vi "RTB.vi"() -> ()   [LabVIEW 2019]
uses:
  <vilib>/Analysis/NI_AALPro.lvlib
  <vilib>/Analysis/NI_AALBase.lvlib
panel:
  out "mean":dbl
  in  "x":dbl=50.0 format="%#_13g"
  out "Lower 2":dbl
  out "Upper 2":dbl
  out "Boolean 3":bool
  out "output array 2":dbl[](array[numeric])
  out "size(s) 2":dbl
  in  "OK Button":bool
  out "Waveform Graph":dbl[](graph)
  out "initialized array":dbl[](array[numeric])
  in  "stop":bool
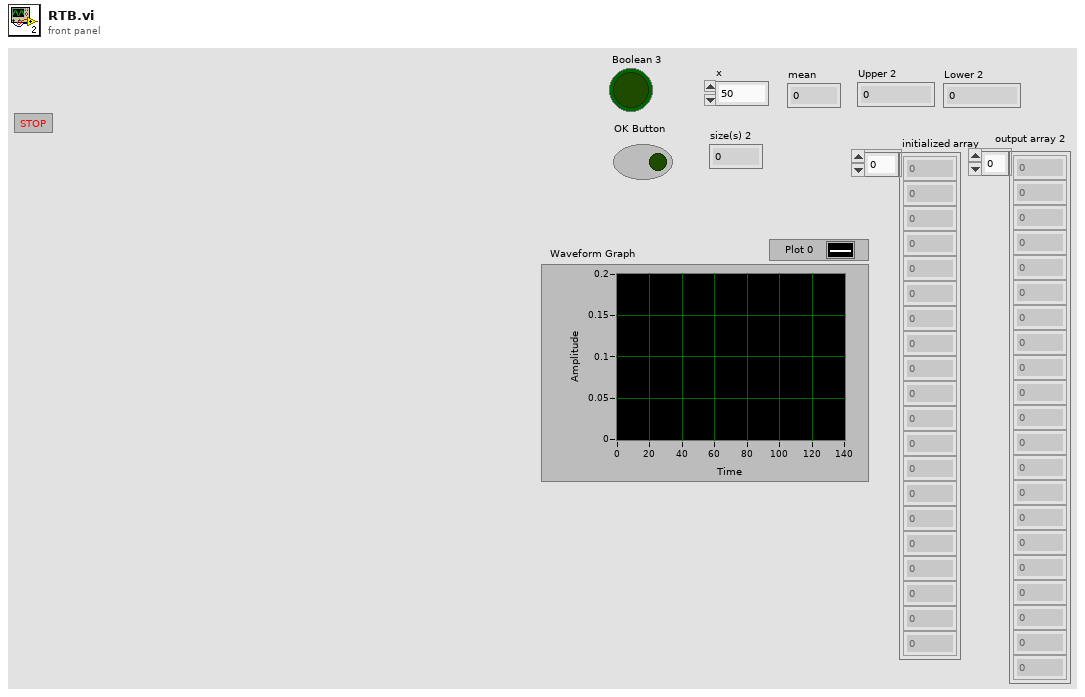
[diagram p1: front panel]
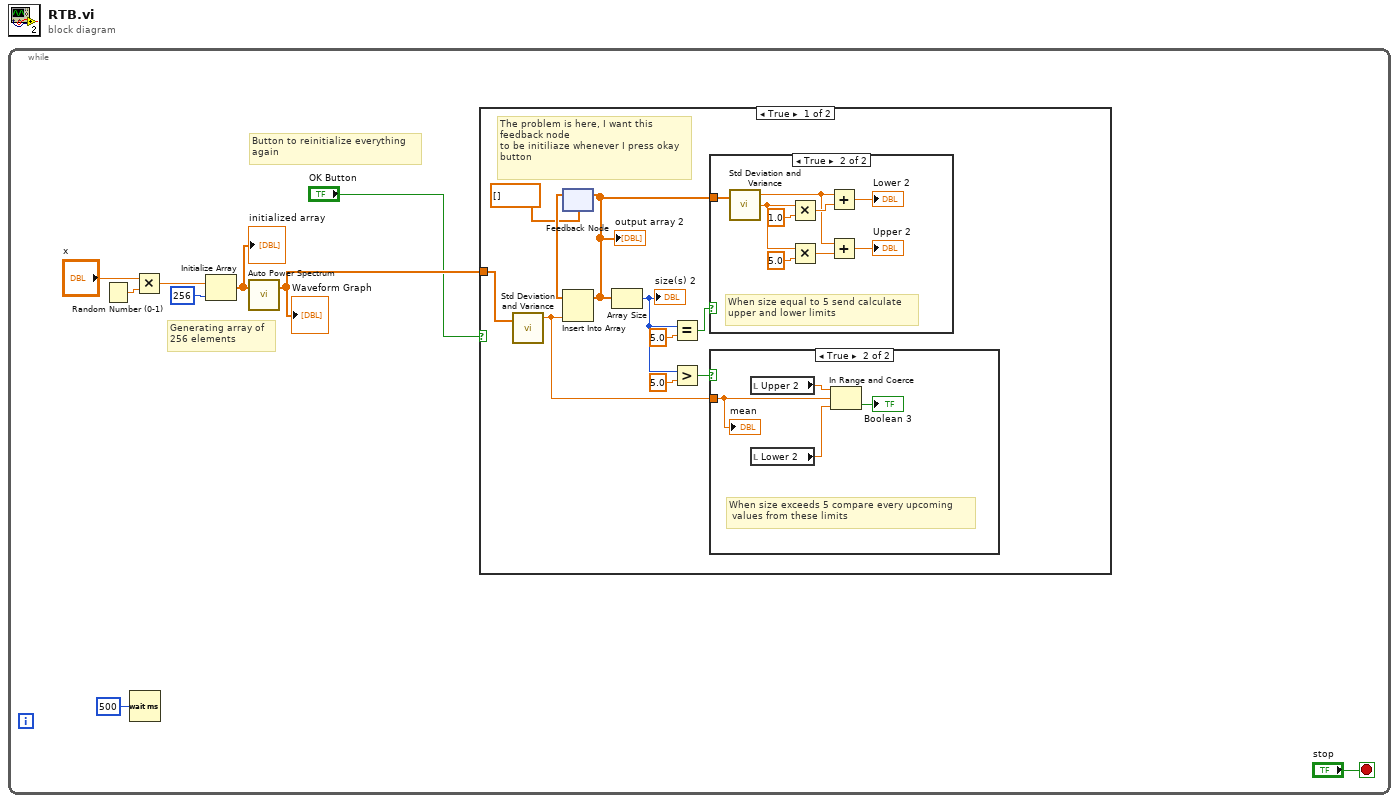
[diagram p0: block diagram]
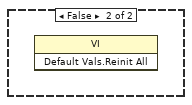
[diagram p4: hidden frame]
diagram:
  n1 = while {
    stop <- "stop" stop-if-true
    # "Generating array of \n256 elements"
    # "Button to reinitialize everything \nagain"
    n2 = Random Number (0-1)() -> (number: 0 to 1=w3:dbl)
    n3 = Wait (ms)(milliseconds to wait=u32 500) -> ()  [unwired: 1 out]
    n4 = Multiply(x="x", y=w3) -> (x*y=w1:dbl)
    n5 = Initialize Array(w1, 256 ("dimension size")) -> (w7:dbl[])
    "initialized array" <- w7
    n6 = call <vilib>:"Auto Power Spectrum.vi"("Signal (V)"=w7) -> ("Power Spectrum (V^2 rms)"=w6:dbl[])  [unwired: 1 in, 1 out]
    "Waveform Graph" <- w6
    n7 = case shown="True" "OK Button" {
      tunnel: w6 -> [w19 _]
      frame True {
        # "The problem is here, I want this feedback node \nto be initiliaze whenever I press okay button"
        n8 = call <vilib>:"Std Deviation and Variance.vi"("X"=w19) -> ("mean"=w16:dbl)  [unwired: 1 in, 2 out]
        n9 = feedback #1(dbl[] []) -> (w11:dbl[])
        n10 = Insert Into Array(array=w11, new element=w16) -> (w12:dbl[])  [unwired: 1 in]
        "output array 2" <- w12
        n11 = feedback-in #1(w12) -> ()
        n12 = Array Size(array=w12) -> (size(s)=w13:i32)
        "size(s) 2" <- w13
        n13 = Equal?(x=w13, y=5.0) -> (x = y?=w17:bool)
        n14 = Greater?(x=w13, y=5.0) -> (0:w15:bool)
        n15 = case shown="True" w17 {
          tunnel: w12 -> [_ w25]
          frame False {
          }
          frame True {
            # "When size equal to 5 send calculate \nupper and lower limits"
            n16 = call <vilib>:"Std Deviation and Variance.vi"("X"=w25) -> ("mean"=w27:dbl, "standard deviation"=w28:dbl)  [unwired: 1 in, 1 out]
            n17 = Multiply(x=w28, y=1.0) -> (x*y=w31:dbl)
            n18 = Multiply(x=w28, y=5.0) -> (x*y=w29:dbl)
            n19 = Add(x=w27, y=w31) -> (x+y=→"Lower 2":dbl)
            n20 = Add(x=w27, y=w29) -> (x+y=→"Upper 2":dbl)
          }
        }
        n21 = case shown="True" w15 {
          tunnel: w16 -> [_ w20]
          frame False {
          }
          frame True {
            # "When size exceeds 5 compare every upcoming\n values from these limits"
            n22 = local read "Upper 2"() -> (w23:dbl)
            n23 = local read "Lower 2"() -> (w22:dbl)
            n24 = In Range and Coerce(upper limit=w23, x=w20, lower limit=w22) -> (In Range?=→"Boolean 3":bool)  [unwired: 1 out]
            "mean" <- w20
          }
        }
      }
      frame False {
        n25 = invoke class="VI" method="Default Vals.Reinit All"() -> ()  [unwired: 3 in, 3 out]
      }
    }
  }
